vi "SELECT ITEM ARCHIVE COLUMNS.vi"(8 "Search Database Results":refnum<vi>, 9 "DATA IN":string[][](array[string]), 11 "Inventory Archive Column Selector":T1) -> (1 "HEADERS OUT":string[](array[string]), 3 "DATA OUT":string[][](array[string]))   [LabVIEW 2019]
uses:
  Controls/Column Names/Inventory Archive Column Names.ctl
  <vilib>/Utility/miscctls.llb/LVRowAndColumnTypeDef.ctl
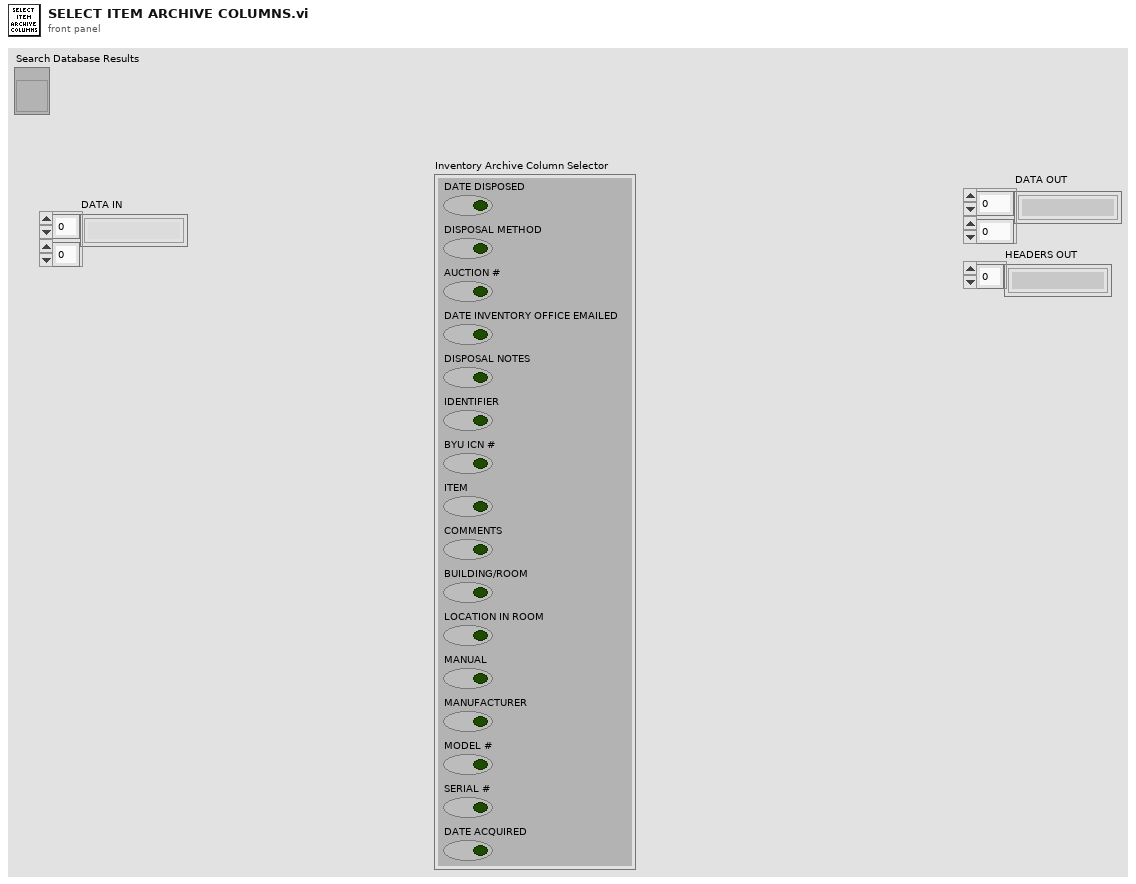
[diagram p1: front panel]
types:
  T1 = cluster{"DATE DISPOSED":bool, "DISPOSAL METHOD":bool, "AUCTION #":bool, "DATE INVENTORY OFFICE EMAILED":bool, "DISPOSAL NOTES":bool, "IDENTIFIER":bool, "BYU ICN #":bool, "ITEM":bool, "COMMENTS":bool, "BUILDING/ROOM":bool, "LOCATION IN ROOM":bool, "MANUAL":bool, "MANUFACTURER":bool, "MODEL #":bool, "SERIAL #":bool, "DATE ACQUIRED":bool}
  T2 = typedef "Inventory Archive Column Names.ctl" = string[]
  T3 = typedef "LVRowAndColumnTypeDef.ctl" = cluster{"Row":i32, "Column":i32}
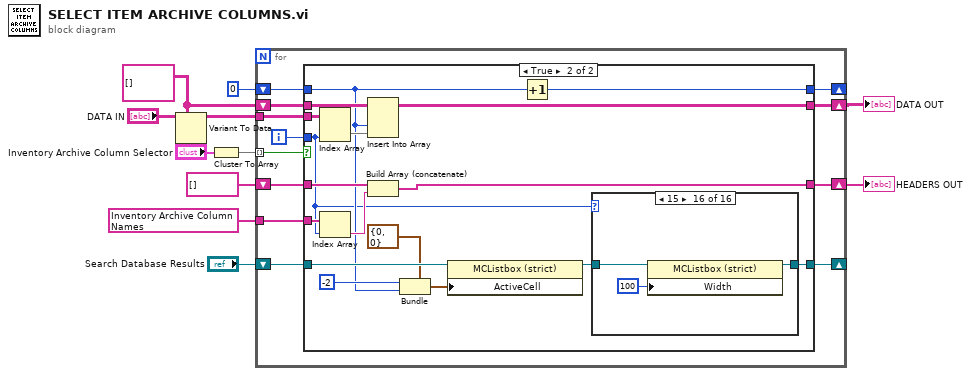
[diagram p0: block diagram]
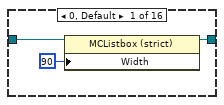
[diagram p3: hidden frame]
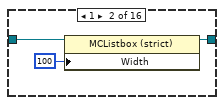
[diagram p4: hidden frame]
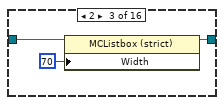
[diagram p5: hidden frame]
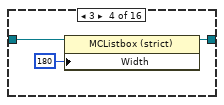
[diagram p6: hidden frame]
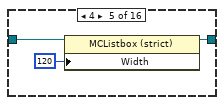
[diagram p7: hidden frame]
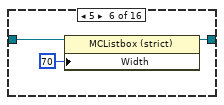
[diagram p8: hidden frame]
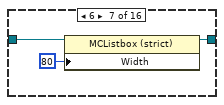
[diagram p9: hidden frame]
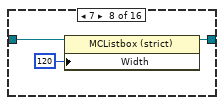
[diagram p10: hidden frame]
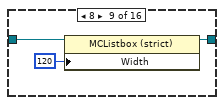
[diagram p11: hidden frame]
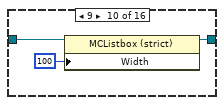
[diagram p12: hidden frame]
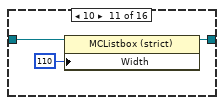
[diagram p13: hidden frame]
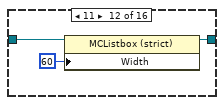
[diagram p14: hidden frame]
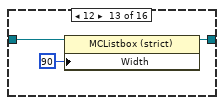
[diagram p15: hidden frame]
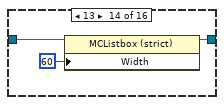
[diagram p16: hidden frame]
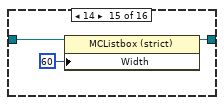
[diagram p17: hidden frame]
diagram:
  w7 = string[][] [] ("DATA OUT")
  n1 = Variant To Data(type=w7, Variant="DATA IN") -> (data=w6:string[][])  [unwired: 1 in, 1 out]
  n2 = Cluster To Array(cluster="Inventory Archive Column Selector") -> (array=w5:bool[])
  n3 = for {
    tunnel: w5 -> [w21] mode=indexing
    tunnel: w6 -> [w23]
    shift-right: [w17] -> w10
    shift-left: w7 -> [w20]
    shift-right: [w18] -> _
    shift-left: 0 -> [w19]
    tunnel: T2 ["Date Disposed", "Disposal Method", "Auction #", "Date Inventory Office Emailed", "Disposal Notes", "ME #/ ID #", "BYU ICN #", "Item Description", "Comments", "Building/Room", "Location in Room", "Manual", "Manufacturer", "Model #", "Serial #", "Date Acquired"] ("INVENTORY ARCHIVE COLUMN NAMES") -> [w16]
    shift-right: [w14] -> w9
    shift-left: string[] [] ("DATA OUT") -> [w15]
    shift-right: [w12] -> _
    shift-left: "Search Database Results" -> [w13]
    i -> [w22]
    n4 = case shown="True" w21 {
      tunnel: w23 -> [_ w44]
      tunnel: w22 -> [_ w30]
      tunnel: w20 -> [w26 w43]
      tunnel: w19 -> [w27 w31]
      tunnel: [w27 w41] -> w18
      tunnel: [w26 w40] -> w17
      tunnel: w16 -> [_ w39]
      tunnel: w15 -> [w25 w38]
      tunnel: [w25 w36] -> w14
      tunnel: w13 -> [w24 w35]
      tunnel: [w24 w28] -> w12
      frame False {
      }
      frame True {
        n5 = Index Array(array=w44, index (col)=w30) -> (element=w42:string[])  [unwired: 1 in]
        n6 = Index Array(array=w39, index=w30) -> (element=w37:string)
        n7 = Insert Into Array(array=w43, index (col)=w31, new element=w42) -> (w40:string[][])  [unwired: 1 in]
        n8 = Build Array (concatenate)(w38, w37) -> (w36:string[])
        n9 = Bundle(cluster=T3 {"Row"=0, "Column"=0} ("Active Cell:Active Cell"), "Row"=-2, "Column"=w31) -> (w33:T3)
        n10 = property class="MCListbox (strict)"(reference=w35, "ActiveCell"=w33) -> (reference out=w29:refnum<vi>)  [unwired: 1 in, 1 out]
        n11 = Increment(x=w31) -> (x+1=w41:i32)
        n12 = case shown="15" w30 {
          tunnel: w29 -> [w47 w50 w53 w56 w59 w62 w65 w68 w71 w74 w77 w80 w83 w86 w89 w92]
          tunnel: [w46 w49 w52 w55 w58 w61 w64 w67 w70 w73 w76 w79 w82 w85 w88 w91] -> w28
          frame 0, Default {
            n13 = property class="MCListbox (strict)"(reference=w47, "Width"=u32 90 ("Active Cell:Cell Size:Width")) -> (reference out=w46:refnum<vi>)  [unwired: 1 in, 1 out]
          }
          frame 1 {
            n14 = property class="MCListbox (strict)"(reference=w50, "Width"=u32 100 ("Active Cell:Cell Size:Width")) -> (reference out=w49:refnum<vi>)  [unwired: 1 in, 1 out]
          }
          frame 2 {
            n15 = property class="MCListbox (strict)"(reference=w53, "Width"=u32 70 ("Active Cell:Cell Size:Width")) -> (reference out=w52:refnum<vi>)  [unwired: 1 in, 1 out]
          }
          frame 3 {
            n16 = property class="MCListbox (strict)"(reference=w56, "Width"=u32 180 ("Active Cell:Cell Size:Width")) -> (reference out=w55:refnum<vi>)  [unwired: 1 in, 1 out]
          }
          frame 4 {
            n17 = property class="MCListbox (strict)"(reference=w59, "Width"=u32 120 ("Active Cell:Cell Size:Width")) -> (reference out=w58:refnum<vi>)  [unwired: 1 in, 1 out]
          }
          frame 5 {
            n18 = property class="MCListbox (strict)"(reference=w62, "Width"=u32 70 ("Active Cell:Cell Size:Width")) -> (reference out=w61:refnum<vi>)  [unwired: 1 in, 1 out]
          }
          frame 6 {
            n19 = property class="MCListbox (strict)"(reference=w65, "Width"=u32 80 ("Active Cell:Cell Size:Width")) -> (reference out=w64:refnum<vi>)  [unwired: 1 in, 1 out]
          }
          frame 7 {
            n20 = property class="MCListbox (strict)"(reference=w68, "Width"=u32 120 ("Active Cell:Cell Size:Width")) -> (reference out=w67:refnum<vi>)  [unwired: 1 in, 1 out]
          }
          frame 8 {
            n21 = property class="MCListbox (strict)"(reference=w71, "Width"=u32 120 ("Active Cell:Cell Size:Width")) -> (reference out=w70:refnum<vi>)  [unwired: 1 in, 1 out]
          }
          frame 9 {
            n22 = property class="MCListbox (strict)"(reference=w74, "Width"=u32 100 ("Active Cell:Cell Size:Width")) -> (reference out=w73:refnum<vi>)  [unwired: 1 in, 1 out]
          }
          frame 10 {
            n23 = property class="MCListbox (strict)"(reference=w77, "Width"=u32 110 ("Active Cell:Cell Size:Width")) -> (reference out=w76:refnum<vi>)  [unwired: 1 in, 1 out]
          }
          frame 11 {
            n24 = property class="MCListbox (strict)"(reference=w80, "Width"=u32 60 ("Active Cell:Cell Size:Width")) -> (reference out=w79:refnum<vi>)  [unwired: 1 in, 1 out]
          }
          frame 12 {
            n25 = property class="MCListbox (strict)"(reference=w83, "Width"=u32 90 ("Active Cell:Cell Size:Width")) -> (reference out=w82:refnum<vi>)  [unwired: 1 in, 1 out]
          }
          frame 13 {
            n26 = property class="MCListbox (strict)"(reference=w86, "Width"=u32 60 ("Active Cell:Cell Size:Width")) -> (reference out=w85:refnum<vi>)  [unwired: 1 in, 1 out]
          }
          frame 14 {
            n27 = property class="MCListbox (strict)"(reference=w89, "Width"=u32 60 ("Active Cell:Cell Size:Width")) -> (reference out=w88:refnum<vi>)  [unwired: 1 in, 1 out]
          }
          frame 15 {
            n28 = property class="MCListbox (strict)"(reference=w92, "Width"=u32 100 ("Active Cell:Cell Size:Width")) -> (reference out=w91:refnum<vi>)  [unwired: 1 in, 1 out]
          }
        }
      }
    }
  }
  "DATA OUT" <- w10
  "HEADERS OUT" <- w9
